vi "Close Log File Instance.vi"(8 "error in (no error)":errorcluster, 11 "Segmented Log in":refnum<class "Segmented Log.lvclass">) -> (0 "error out":errorcluster, 3 "Segmented Log out":refnum<class "Segmented Log.lvclass">)   [LabVIEW 2015, in "Segmented Log.lvclass"]
doc: "Close the file and set it to read-only if specified. Notify any listeners that this log file has been closed. Add the file to the list of log files if not already added."
uses:
  Segmented Log.lvclass
  Segmented Log.lvclass/Segmented Log.ctl
  Log Files/Log File/Log File.lvclass/Log File.ctl
  Log Files/TDMS Log File/TDMS Log File.lvclass/TDMS Log File.ctl
  Log Files/Text Log File/Text Log File.lvclass/Text Log File.ctl
  Log Files/TDMS Log File/Close TDMS Log File.vi
  Log Files/Text Log File/Close Text Log File.vi
  Log Files/Text Log File/Text Log File.lvclass
  Log Files/TDMS Log File/TDMS Log File.lvclass
  Log Files/Log File/Log File.lvclass
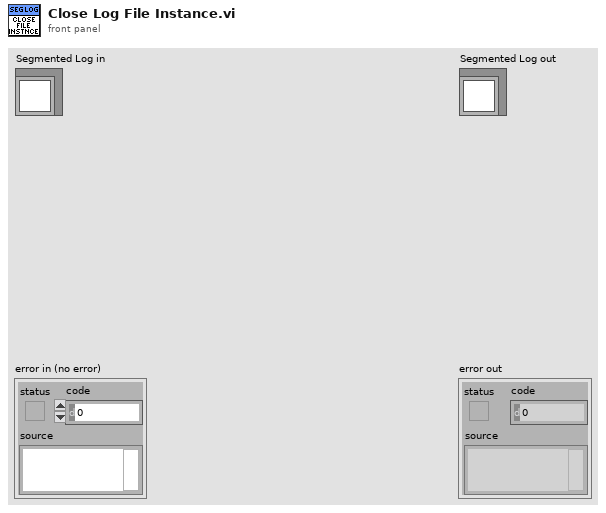
[diagram p1: front panel]
types:
  T1 = typedef "Segmented Log.lvclass/File Close Event Registration.ctl" = cluster{"Callback":refnum<vi>, "User Data":variant}
  T2 = typedef "Segmented Log.lvclass/Segmented Log Complete Event Registration.ctl" = cluster{"Callback":refnum<vi>, "User Data":variant}
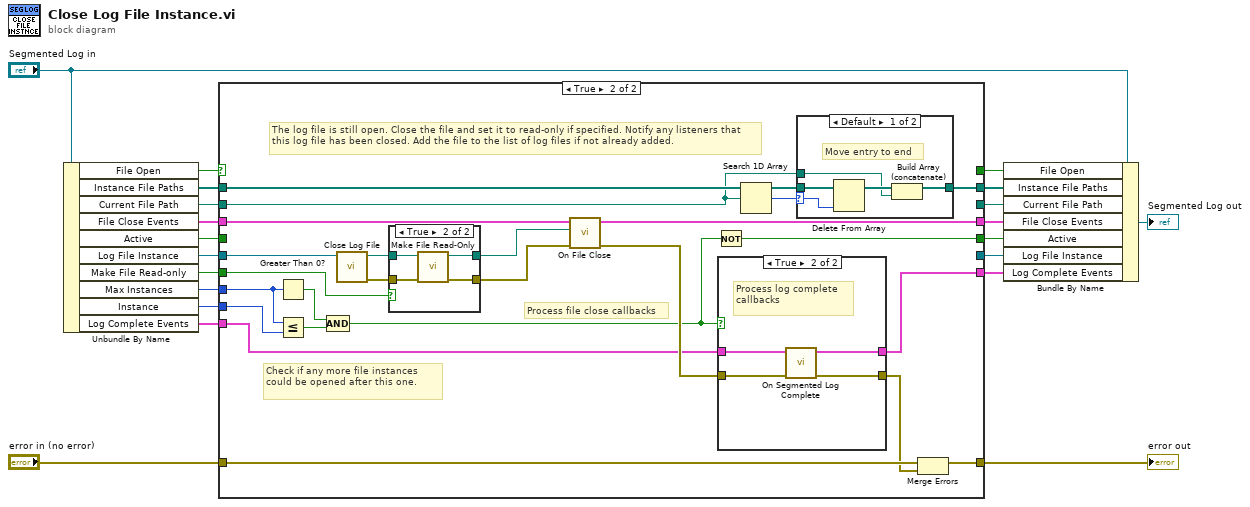
[diagram p0: block diagram]
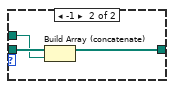
[diagram p3: hidden frame]
diagram:
  n1 = Unbundle By Name("Segmented Log in") -> ("File Open"=w12:bool, "Instance File Paths"=w17:path[], "Current File Path"=w16:path, "File Close Events"=w19:T1[], "Active"=w7:bool, "Log File Instance"=w13:refnum<class "Log File.lvclass">, "Make File Read-only"=w4:bool, "Max Instances"=w6:i32, "Instance"=w5:i32, "Log Complete Events"=w2:T2[])
  n2 = case shown="True" w12 {
    selector: w12 -> [w26 _]
    tunnel: w13 -> [w23 w52]
    tunnel: w19 -> [w29 w36]
    tunnel: [w29 w35] -> w18
    tunnel: [w24 w38] -> w8
    tunnel: w17 -> [w28 w32]
    tunnel: w16 -> [w27 w30]
    tunnel: [w28 w49] -> w15
    tunnel: [w27 _] -> w14
    tunnel: [w26 _] -> w11
    tunnel: "error in (no error)" -> [w25 w48]
    tunnel: [w25 w47] -> w9
    tunnel: w7 -> [w24 _]
    tunnel: w6 -> [_ w44]
    tunnel: w5 -> [_ w43]
    tunnel: w4 -> [_ w42]
    tunnel: [w23 _] -> w3
    tunnel: w2 -> [w22 w41]
    tunnel: [w22 w40] -> w1
    frame False {
    }
    frame True {
      # "Process file close callbacks"
      # "Check if any more file instances could be opened after this one."
      # "The log file is still open. Close the file and set it to read-only if specified. Notify any listeners that this log file has been closed. Add the file to the list of log files if not already added."
      n3 = Greater Than 0?(x=w44) -> (x > 0?=w46:bool)
      n4 = Less Or Equal?(x=w44, y=w43) -> (x <= y?=w45:bool)
      n5 = Compound Arithmetic op=AND(w46, w45) -> (w37:bool)
      n6 = call "Close Log File.vi"("Log File in"=w52) -> ("error out"=w51:errorcluster, "File Path"=w50:path)  [unwired: 9 in]
      n7 = case shown="True" w42 {
        tunnel: [w69 w71] -> w33
        tunnel: w51 -> [w69 w72]
        tunnel: w50 -> [w68 w73]
        tunnel: [w68 w70] -> w34
        frame False {
        }
        frame True {
          n8 = call "Make File Read-Only.vi"("error in (no error)"=w72, "File Path in"=w73) -> ("error out"=w71:errorcluster, "File Path out"=w70:path)  [unwired: 8 in]
        }
      }
      n9 = call "On File Close.vi"("error in (no error)"=w33, "Path"=w34, "File Close Event Registrations in"=w36) -> ("error out"=w53:errorcluster, "File Close Event Registrations out"=w35:T1[])  [unwired: 7 in]
      n10 = Not(x=w37) -> (.not. x?=w38:bool)
      n11 = case shown="True" w37 {
        tunnel: w41 -> [w63 w67]
        tunnel: [w63 w66] -> w40
        tunnel: w53 -> [w62 w65]
        tunnel: [w62 w64] -> w39
        frame False {
        }
        frame True {
          # "Process log complete callbacks"
          n12 = call "On Segmented Log Complete.vi"("error in (no error)"=w65, "File Open Event Registrations in"=w67) -> ("error out"=w64:errorcluster, "File Open Event Registrations out"=w66:T2[])  [unwired: 8 in]
        }
      }
      n13 = Search 1D Array(1D array=w32, element=w30) -> (index of element=w31:i32)  [unwired: 1 in]
      n14 = case shown="Default" w31 {
        selector: w31 -> [w57 _]
        tunnel: [w54 w61] -> w49
        tunnel: w32 -> [w58 w60]
        tunnel: w30 -> [w55 w59]
        frame Default {
          # "Move entry to end"
          n15 = Delete From Array(array=w58, index=w57) -> (array with subset deleted=w56:path[])  [unwired: 1 in, 1 out]
          n16 = Build Array (concatenate)(w56, w55) -> (w54:path[])
        }
        frame -1 {
          n17 = Build Array (concatenate)(w60, w59) -> (w61:path[])
        }
      }
      n18 = Merge Errors(w48, w39) -> (w47:errorcluster)
    }
  }
  "error out" <- w9
  n19 = Bundle By Name(cluster="Segmented Log in", "File Open"=w11, "Instance File Paths"=w15, "Current File Path"=w14, "File Close Events"=w18, "Active"=w8, "Log File Instance"=w3, "Log Complete Events"=w1) -> (→"Segmented Log out":refnum<class "Segmented Log.lvclass">)
